vi "v_2.vi"() -> ()   [LabVIEW 2014]
uses:
  <vilib>/LabVIEW Interface for Arduino/Type Defs/Pin Mode.ctl
  <vilib>/LabVIEW Interface for Arduino/LabVIEW Interface for Arduino.lvlib
panel:
  in  "VISA resource":refnum<visa-resource-name>
  in  "stop":bool
  in  "Forward":bool
  in  "Backward":bool
  in  "Dial":dbl(knob) scale=0.0..255.0
  out "Speed":dbl(knob) scale=0.0..100.0
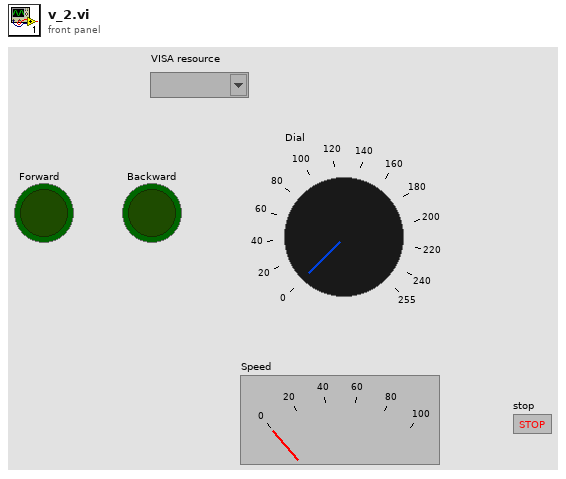
[diagram p1: front panel]
types:
  T1 = typedef "LabVIEW Interface for Arduino.lvlib/Arduino Resource.ctl" = cluster{"VISA resource":refnum<visa-resource-name>, "Board Type":T2, "Connection Type":enum8{"USB / Serial"}, "Bytes Per Packet (15)":u8}
  T2 = typedef "LabVIEW Interface for Arduino.lvlib/Board Type.ctl" = enum16{"Uno", "Dimuelanove w/Atmega 328", "Mega 2560"}
  T3 = typedef "LabVIEW Interface for Arduino.lvlib/Pin Mode.ctl" = enum8{"Input", "Output"}
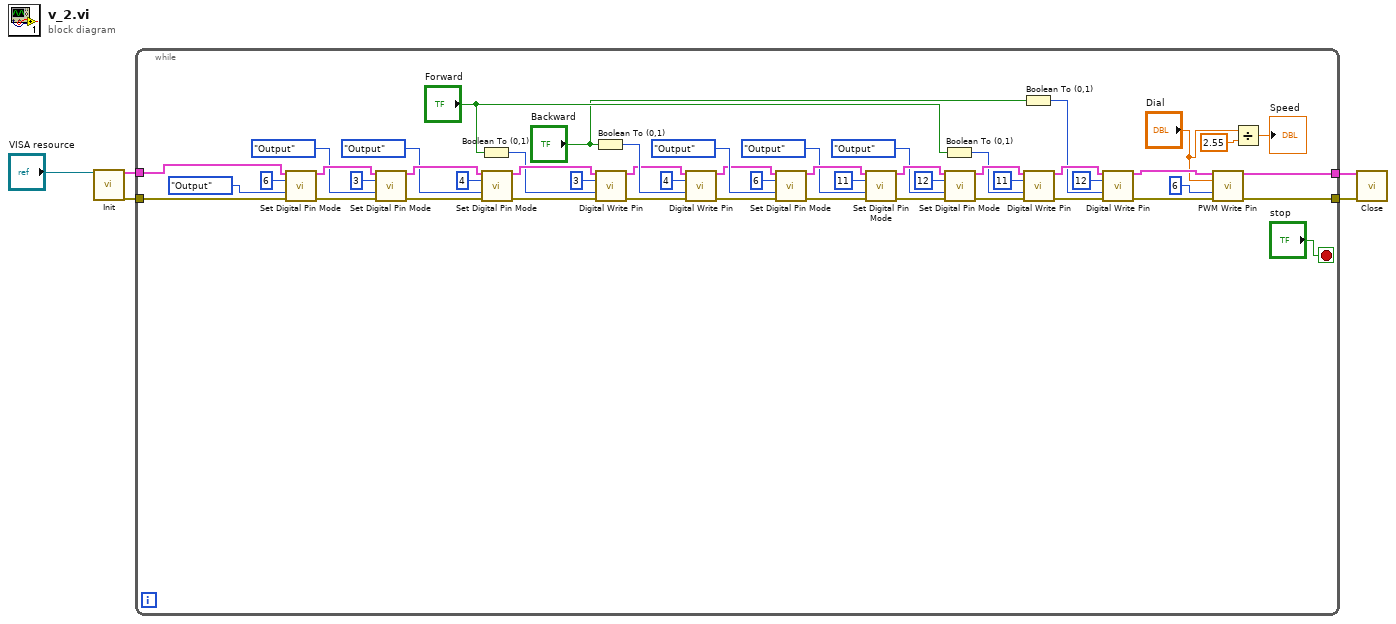
[diagram p0: block diagram]
diagram:
  n1 = call <vilib>:"Init.vi"("VISA resource"="VISA resource") -> ("Arduino Resource"=w3:T1, "error out"=w2:errorcluster)  [unwired: 17 in]
  n2 = while {
    tunnel: w3 -> [w56]
    tunnel: w2 -> [w55]
    tunnel: [w12] -> w5
    tunnel: [w11] -> w4
    stop <- "stop" stop-if-true
    n3 = call <vilib>:"Set Digital Pin Mode.vi"("Arduino Resource"=w56, "Digital I/O Pin"=u8 6, "Pin Mode (Input)"=Pin_Mode."Output", "error in"=w55) -> ("Arduino Resource"=w51:T1, "error out"=w50:errorcluster)  [unwired: 10 in]
    n4 = call <vilib>:"Set Digital Pin Mode.vi"("Arduino Resource"=w51, "Digital I/O Pin"=u8 3, "Pin Mode (Input)"=Pin_Mode."Output", "error in"=w50) -> ("Arduino Resource"=w47:T1, "error out"=w46:errorcluster)  [unwired: 10 in]
    n5 = Boolean To (0,1)(Boolean="Forward") -> (0, 1=w40:i16)
    n6 = call <vilib>:"Set Digital Pin Mode.vi"("Arduino Resource"=w47, "Digital I/O Pin"=u8 4, "Pin Mode (Input)"=Pin_Mode."Output", "error in"=w46) -> ("Arduino Resource"=w43:T1, "error out"=w42:errorcluster)  [unwired: 10 in]
    n7 = Boolean To (0,1)(Boolean="Backward") -> (0, 1=w38:i16)
    n8 = call <vilib>:"Digital Write Pin.vi"("Arduino Resource"=w43, "Digital I/O Pin (0)"=u8 3, "Value (0)"=w40, "error in"=w42) -> ("Arduino Resource"=w37:T1, "error out"=w36:errorcluster)  [unwired: 10 in]
    n9 = call <vilib>:"Digital Write Pin.vi"("Arduino Resource"=w37, "Digital I/O Pin (0)"=u8 4, "Value (0)"=w38, "error in"=w36) -> ("Arduino Resource"=w16:T1, "error out"=w15:errorcluster)  [unwired: 10 in]
    n10 = call <vilib>:"Set Digital Pin Mode.vi"("Arduino Resource"=w16, "Digital I/O Pin"=u8 6, "Pin Mode (Input)"=Pin_Mode."Output", "error in"=w15) -> ("Arduino Resource"=w30:T1, "error out"=w29:errorcluster)  [unwired: 10 in]
    n11 = call <vilib>:"Set Digital Pin Mode.vi"("Arduino Resource"=w30, "Digital I/O Pin"=u8 11, "Pin Mode (Input)"=Pin_Mode."Output", "error in"=w29) -> ("Arduino Resource"=w26:T1, "error out"=w25:errorcluster)  [unwired: 10 in]
    n12 = Boolean To (0,1)(Boolean="Forward") -> (0, 1=w6:i16)
    n13 = call <vilib>:"Set Digital Pin Mode.vi"("Arduino Resource"=w26, "Digital I/O Pin"=u8 12, "Pin Mode (Input)"=Pin_Mode."Output", "error in"=w25) -> ("Arduino Resource"=w22:T1, "error out"=w21:errorcluster)  [unwired: 10 in]
    n14 = Boolean To (0,1)(Boolean="Backward") -> (0, 1=w7:i16)
    n15 = call <vilib>:"Digital Write Pin.vi"("Arduino Resource"=w22, "Digital I/O Pin (0)"=u8 11, "Value (0)"=w6, "error in"=w21) -> ("Arduino Resource"=w18:T1, "error out"=w17:errorcluster)  [unwired: 10 in]
    n16 = call <vilib>:"Digital Write Pin.vi"("Arduino Resource"=w18, "Digital I/O Pin (0)"=u8 12, "Value (0)"=w7, "error in"=w17) -> ("Arduino Resource"=w14:T1, "error out"=w13:errorcluster)  [unwired: 10 in]
    n17 = call <vilib>:"PWM Write Pin.vi"("Arduino Resource"=w14, "Duty Cycle (0 - 255)"="Dial", "PWM Pin (3)"=u8 6, "error in"=w13) -> ("Arduino Resource"=w12:T1, "error out"=w11:errorcluster)  [unwired: 10 in]
    n18 = Divide(x="Dial", y=2.55) -> (x/y=→"Speed":dbl)
  }
  n19 = call <vilib>:"Close.vi"("Arduino Resource"=w5, "error in"=w4) -> ()  [unwired: 13 in, 1 out]
